vi "Calc Type.vi"(11 "Min Calc in":refnum<class "Min Calc.lvclass">) -> (2 "Calc Type":string)   [LabVIEW 2020, in "VolatusCalcs.lvlib" / "Min Calc.lvclass"]
uses:
  Min Calc.lvclass
  Min Calc.lvclass/Min Calc.ctl
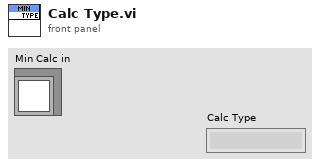
[diagram p1: front panel]
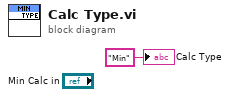
[diagram p0: block diagram]
diagram:
  "Calc Type" <- "Min" ("Calc Type")
